vi "Write Time Stamp.vi"(8 "error in (no error)":errorcluster, 10 "Time Stamp":timestamp, 11 "FeedItem.lvclass in":refnum<class "FeedItem.lvclass">) -> (0 "error out":errorcluster, 3 "FeedItem.lvclass out":refnum<class "FeedItem.lvclass">)   [LabVIEW 2017, in "FeedItem.lvclass"]
uses:
  <vilib>/NI_RSS/FeedItem/FeedItem.lvclass
  <vilib>/NI_RSS/FeedItem/FeedItem.lvclass/FeedItem.ctl
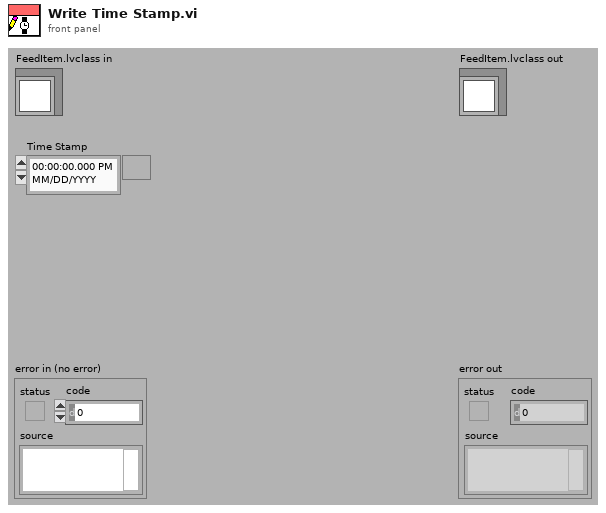
[diagram p1: front panel]
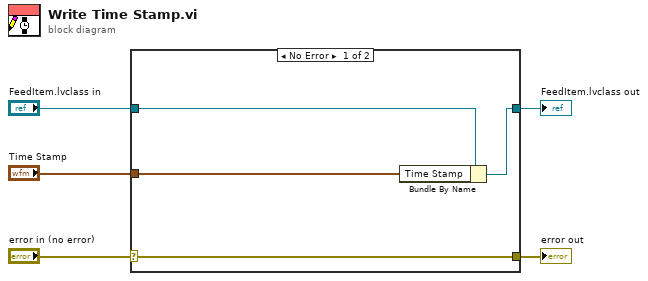
[diagram p0: block diagram]
diagram:
  n1 = case shown="No Error" "error in (no error)" {
    selector: "error in (no error)" -> [w9 w10]
    tunnel: [w9 w10] -> w4
    tunnel: [w7 w11] -> w2
    tunnel: "FeedItem.lvclass in" -> [w8 w11]
    tunnel: "Time Stamp" -> [w6 _]
    frame No Error {
      n2 = Bundle By Name(cluster=w8, "Time Stamp"=w6) -> (w7:refnum<class "FeedItem.lvclass">)
    }
    frame Error {
    }
  }
  "error out" <- w4
  "FeedItem.lvclass out" <- w2
